vi "HXG2saveFGV.vi"(7 "saveFGV":T1, 8 "error in (no error)":errorcluster, 9 "tdms ref In":refnum<k34>, 10 "HX Description":string="HXname", 11 "Capture Data":bool) -> (0 "error out":errorcluster, 1 "Full Path":path, 3 "Saving?":bool, 4 "tdms file out":refnum<k34>, 5 "Partial Path":path)   [LabVIEW 2012]
uses:
  HXG2save.ctl
  <vilib>/Utility/sysdir.llb/System Directory Type.ctl
panel:
  in  "Capture Data 2":bool
  out "Home directory":path
  out "appended path":path
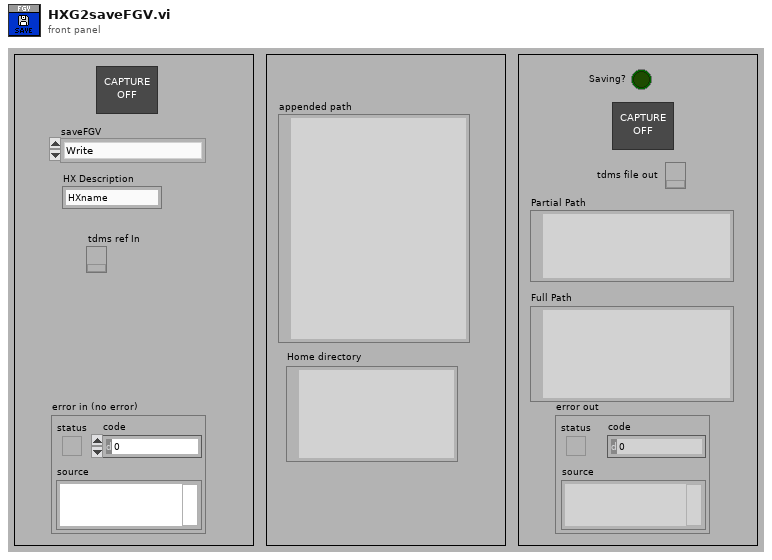
[diagram p1: front panel]
types:
  T1 = typedef "HXG2save.ctl" = enum16{"Write", "Pass", "Initialize", "Kill"}
  T2 = enum16{"open", "open or create", "create or replace", "create", "open (read-only)"}
  T3 = typedef "System Directory Type.ctl" = i32
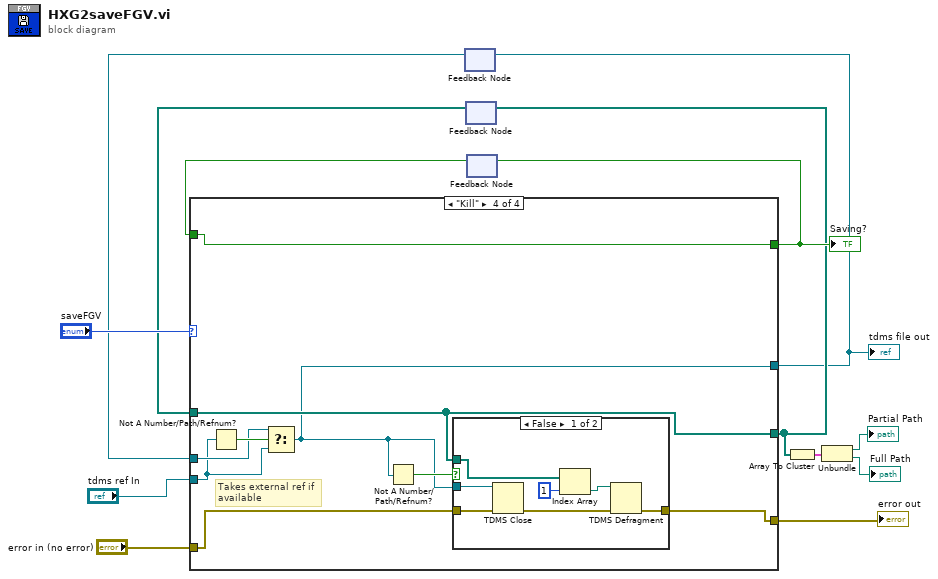
[diagram p0: block diagram]
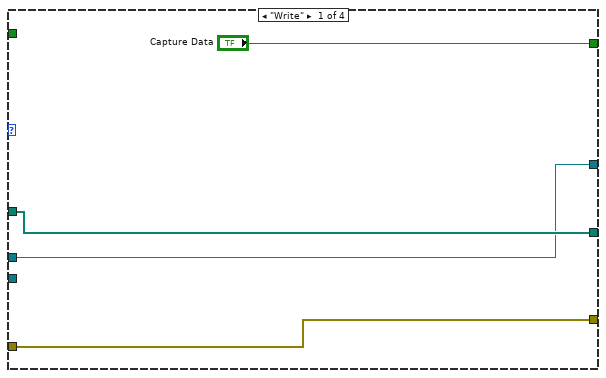
[diagram p2: hidden frame]
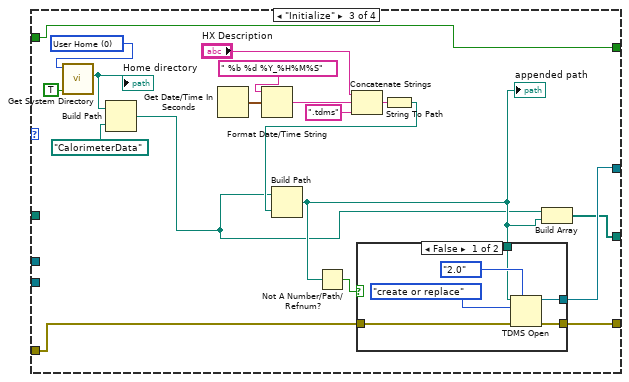
[diagram p4: hidden frame]
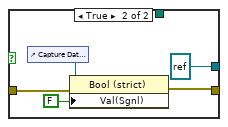
[diagram p5: hidden frame]
diagram:
  n1 = feedback #1() -> (w2:refnum<k34>)  [unwired: 1 in]
  n2 = feedback #2() -> (w4:path[])  [unwired: 1 in]
  n3 = feedback #3() -> (w10:bool)  [unwired: 1 in]
  n4 = case shown="\"Kill\"" "saveFGV" {
    tunnel: "error in (no error)" -> [w17 w20 w27 w59]
    tunnel: [w17 w20 w34 w58] -> w12
    tunnel: ["Capture Data" w21 w33 w60] -> w11
    tunnel: w10 -> [_ w21 w33 w60]
    tunnel: [w15 w19 w25 w56] -> w5
    tunnel: w4 -> [w15 w19 _ w56]
    tunnel: [w14 w18 w32 w52] -> w3
    tunnel: w2 -> [w14 w18 _ w54]
    tunnel: "tdms ref In" -> [_ _ _ w53]
    frame "Write" {
    }
    frame "Pass" {
    }
    frame "Initialize" {
      w30 = T3 0 items=["User Home"=0, "User Desktop"=1, "User Documents"=2, "User Application Data"=3, "User Preferences"=4, "User Temporary"=5, "Public Documents"=6, "Public Application Data"=7, "Public Preferences"=8, "Public Cache"=13, "System Core Libraries"=9, "System Installed Libraries"=10, "Application Files"=11, "Boot Volume Root"=12] ("system directory type")
      n5 = call <vilib>:"Get System Directory.vi"("create directory if not found? (F)"=TRUE, "system directory type"=w30) -> ("system directory"=w29:path)  [unwired: 9 in]
      "Home directory" <- w29
      n6 = Build Path(base path=w29, name or relative path=path "CalorimeterData") -> (appended path=w23:path)
      n7 = Get Date/Time In Seconds() -> (seconds since 1Jan1904=w40:timestamp)
      n8 = Format Date/Time String(time format string (%c)=" %b %d %Y_%H%M%S", seconds (now)=w40) -> (date/time string=w38:string)  [unwired: 1 in]
      n9 = Concatenate Strings("HX Description", w38, ".tdms" ("string")) -> (w36:string)
      n10 = String To Path(string=w36) -> (path=w35:path)
      n11 = Build Path(base path=w23, name or relative path=w35) -> (appended path=w24:path)
      "appended path" <- w24
      n12 = Not A Number/Path/Refnum?(number/path/refnum=w24) -> (NaN/Path/Refnum?=w26:bool)
      n13 = case shown="False" w26 {
        tunnel: w24 -> [w44 _]
        tunnel: [w43 w49] -> w34
        tunnel: [w42 refnum<k34> refnum ("tdms file out")] -> w32
        tunnel: w27 -> [w41 w50]
        frame False {
          n14 = TDMS Open(7:enum16{"1.0", "2.0"}."2.0" ("file format version (2.0)"), 8:w41, 10:T2."create or replace" ("operation (0:open)"), 11:w44) -> (0:w43:errorcluster, 3:w42:refnum<k34>)  [unwired: 2 in]
        }
        frame True {
          n15 = control-ref of="Capture Data 2"() -> (w48:refnum<vi>)
          n16 = property class="Bool (strict)"(reference=w48, error in=w50, "Val(Sgnl)"=FALSE ("Value (Signaling)")) -> (error out=w49:errorcluster)  [unwired: 1 out]
        }
      }
      n17 = Build Array(w23, w24) -> (w25:path[])
    }
    frame "Kill" {
      # "Takes external ref if \navailable"
      n18 = Not A Number/Path/Refnum?(number/path/refnum=w53) -> (NaN/Path/Refnum?=w55:bool)
      n19 = Select(t=w54, s=w55, f=w53) -> (s? t:f=w52:refnum<k34>)
      n20 = Not A Number/Path/Refnum?(number/path/refnum=w52) -> (NaN/Path/Refnum?=w57:bool)
      n21 = case shown="False" w57 {
        tunnel: w52 -> [w67 _]
        tunnel: w59 -> [w66 w68]
        tunnel: [w64 w68] -> w58
        tunnel: w56 -> [w63 _]
        frame False {
          n22 = TDMS Close(8:w66, 11:w67) -> (0:w65:errorcluster)  [unwired: 1 out]
          n23 = Index Array(array=w63, index=1) -> (element=w61:path)
          n24 = TDMS Defragment(4:w65, 7:w61) -> (0:w64:errorcluster)
        }
        frame True {
        }
      }
    }
  }
  "error out" <- w12
  "Saving?" <- w11
  "tdms file out" <- w3
  n25 = feedback-in #1(w3) -> ()
  n26 = feedback-in #2(w5) -> ()
  n27 = feedback-in #3(w11) -> ()
  n28 = Array To Cluster(array=w5) -> (cluster=w6:cluster{"[0]":path, "[1]":path})
  n29 = Unbundle(w6) -> ("[0]"=→"Partial Path":path, "[1]"=→"Full Path":path)
